vi "RealtimeAudioVsTimedAudio.vi"(6 "Recording Duration (s)":dbl=5.0 caption="Duration (s)", 8 "Sample Rate (Hz)":dbl=5.0 caption="Duration (s)", 9 "Waveform Buffer In":dynamicdata(waveform), 10 "Record Sound":bool, 11 "FreeRecord or TimedRecord":bool) -> (1 "FreeRecord Out":dynamicdata(waveform), 2 "RecordingType Status":bool, 3 "Waveform Buffer Storage":dynamicdata(waveform), 4 "Recording Status":bool)   [LabVIEW 2022 SP3]
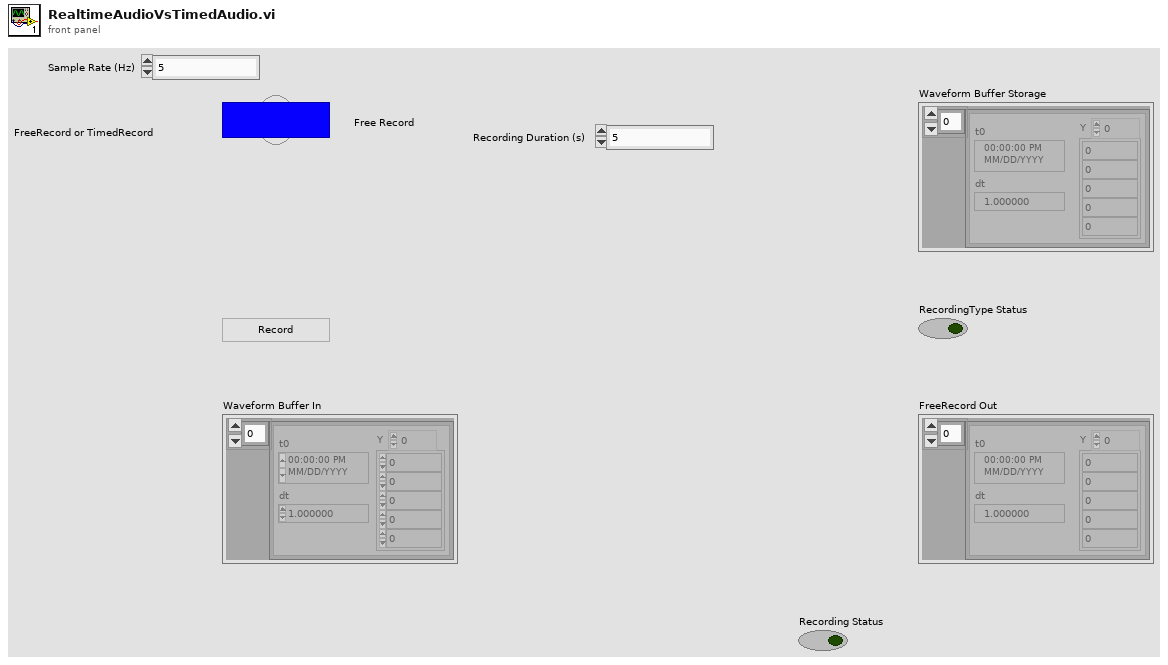
[diagram p1: front panel]
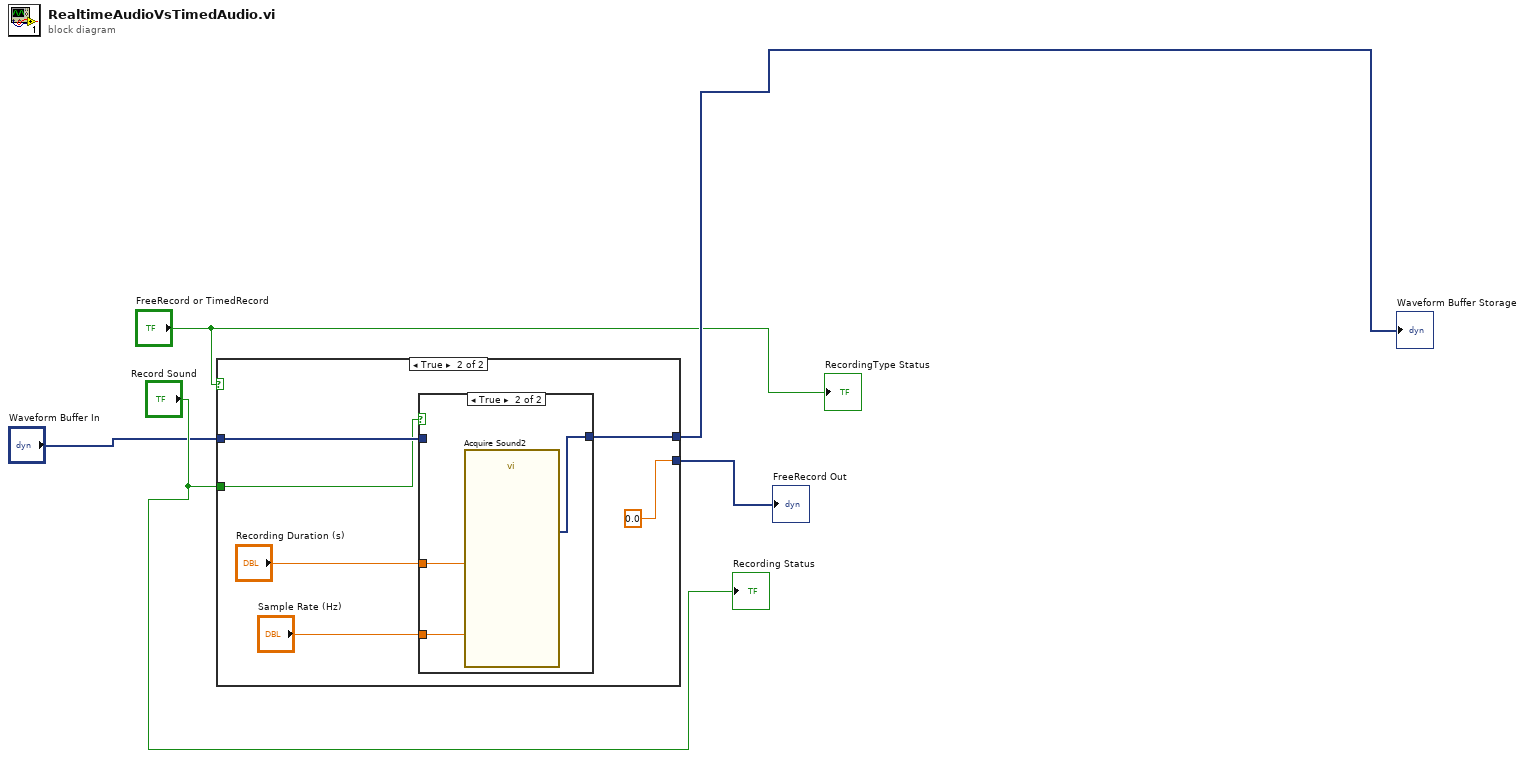
[diagram p0: block diagram]
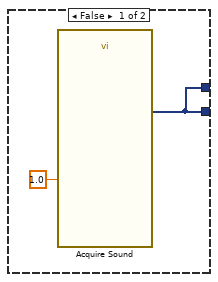
[diagram p2: hidden frame]
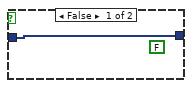
[diagram p3: hidden frame]
diagram:
  n1 = case shown="True" "FreeRecord or TimedRecord" {
    tunnel: [w6 w12] -> w2
    tunnel: "Waveform Buffer In" -> [_ w11]
    tunnel: [w6 0.0] -> w4
    tunnel: "Record Sound" -> [_ w9]
    frame False {
      n2 = call "Acquire Sound"("Duration (s)"=1.0) -> ("Data"=w6:dynamicdata)  [unwired: 17 in, 1 out]
    }
    frame True {
      n3 = case shown="True" w9 {
        tunnel: "Recording Duration (s)" -> [_ w17]
        tunnel: [w14 w16] -> w12
        tunnel: w11 -> [w14 _]
        tunnel: "Sample Rate (Hz)" -> [_ w15]
        frame False {
          (unwired) FALSE
        }
        frame True {
          n4 = call "Acquire Sound2"("Duration (s)"=w17, "Sample rate (Hz)"=w15) -> ("Data"=w16:dynamicdata)  [unwired: 16 in, 1 out]
        }
      }
    }
  }
  "FreeRecord Out" <- w4
  "Waveform Buffer Storage" <- w2
  "Recording Status" <- "Record Sound"
  "RecordingType Status" <- "FreeRecord or TimedRecord"
